vi "close.vi"(8 "error in (no error)":errorcluster, 11 "TC01 in":refnum<class "TC01.lvclass">) -> (0 "error out":errorcluster, 3 "TC01 out":refnum<class "TC01.lvclass">)   [LabVIEW 2025, in "Temperature Sensor.lvlib" / "TC01.lvclass"]
uses:
  TC01.lvclass
  TC01.lvclass/TC01.ctl
  C:/Users/Tyson.Grover/Desktop/Repositories/dqmh-lvoop-template/Libraries/Temperature Sensor/generic-temp-sensor/generic-temp-sensor.lvclass
  C:/Users/Tyson.Grover/Desktop/Repositories/dqmh-lvoop-template/Libraries/Temperature Sensor/Classes/TC01/TC01.lvclass
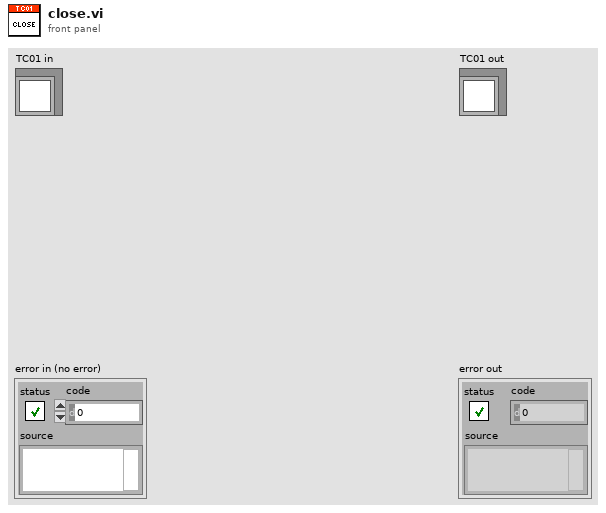
[diagram p1: front panel]
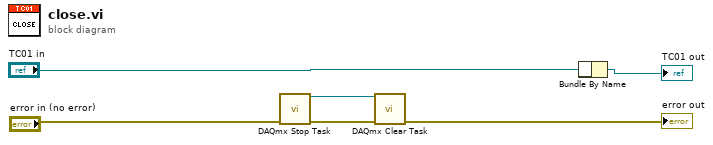
[diagram p0: block diagram]
diagram:
  n1 = call <vilib>:"DAQmx Stop Task.vi"("error in"="error in (no error)") -> ("task out"=w2:refnum<k21>, "error out"=w3:errorcluster)  [unwired: 13 in]
  n2 = call <vilib>:"DAQmx Clear Task.vi"("task in"=w2, "error in"=w3) -> ("error out"=→"error out":errorcluster)  [unwired: 13 in]
  n3 = Bundle By Name(cluster="TC01 in") -> (→"TC01 out":refnum<class "TC01.lvclass">)  [unwired: 1 in]
